vi "Write User Event (Normal).vi"(6 "優先度（通常）":T1, 7 "EvCmd":string, 8 "エラー入力（エラーなし）":errorcluster, 10 "データ":variant, 11 "ユーザイベント入力":refnum<user-event>) -> (0 "エラー出力":errorcluster, 3 "ユーザイベント出力":refnum<user-event>)   [LabVIEW 2014]
uses:
  Ctl/Event Cluster.ctl
  <vilib>/event_ctls.llb/usereventprio.ctl
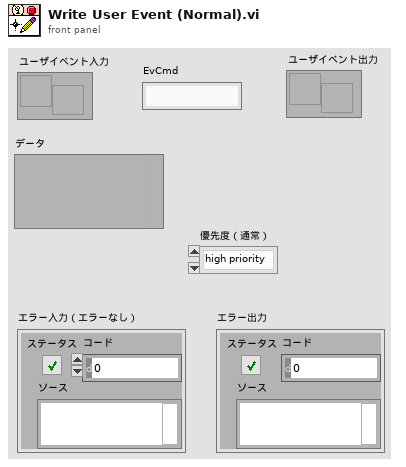
[diagram p1: front panel]
types:
  T1 = typedef "usereventprio.ctl" = enum32{"high priority", "normal priority"}
  T2 = typedef "Event Cluster.ctl" = cluster{"コマンド":string, "バリアント":variant}
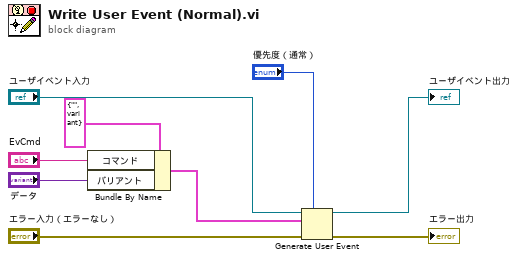
[diagram p0: block diagram]
diagram:
  n1 = Bundle By Name(cluster=T2 {"コマンド"="", "バリアント"=variant} ("Event Cluster"), "コマンド"="EvCmd", "バリアント"="データ") -> (w9:T2)
  n2 = Generate User Event(priority (normal)="優先度（通常）", user event="ユーザイベント入力", event data cluster=w9, error in="エラー入力（エラーなし）") -> (user event out=→"ユーザイベント出力":refnum<user-event>, error out=→"エラー出力":errorcluster)
